vi "Get Epoch Time.vi"() -> (2 "double precision float":dbl format="%#.3f")   [LabVIEW 2021]
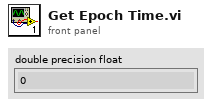
[diagram p1: front panel]
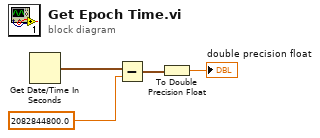
[diagram p0: block diagram]
diagram:
  n1 = Get Date/Time In Seconds() -> (seconds since 1Jan1904=w4:timestamp)
  n2 = Subtract(x=w4, y=2082844800.0) -> (x-y=w2:timestamp)
  n3 = To Double Precision Float(number=w2) -> (double precision float=→"double precision float":dbl)
